vi "WS1050_RFFE_ST Scope Ver1.3.vi"(0 "RFFE PIC":refnum<visa-resource-name>="COM7", 1 "A3643A GPIB":refnum<visa-resource-name>="GPIB1::6::INSTR", 3 "LOT#":string="16VNB", 4 "WAFER#":string="11", 5 "DUT SN":string="SN001R5", 7 "error in (no error)":errorcluster, 8 "Scope USB":refnum<visa-resource-name>="USB0::0x0699::0x0405::C010240::INSTR", 9 "GROUP":string="LEG1-Lord", 12 "path":path=path "C:/Andy/WS1050/ST Test/SN01", 13 "RFT Path":path=path "C:/Andy/WS1050/ST Test", 14 "Start":bool=TRUE, 15 "Stop Loop":bool, 16 "Initilize RFFE ?":bool, 17 "stop":bool=TRUE, 20 "Scope\nSet Up":bool, 22 "Comment":string) -> (10 "RFFE PIC 2":refnum<visa-resource-name>="COM7", 18 "ST Data Out":string[](array[string])=["824.709800E-9", "99.100000E+36", "14.400000E-3", "99.100000E+36", "687.070300E-9", "14.000000E-3", "991.902900E-9", "99.100000E+36", "30.800000E-3", "99.100000E+36", "729.561600E-9", "28.400000E-3", "794.023400E-9", "99.100000E+36", "66.000000E-3", "99.100000E+36", "698.320300E-9", "64.000000E-3", "677.011700E-9", "99.100000E+36", "172.000000E-3", "99.100000E+36", "781.972700E-9", "168.000000E-3", "1.047500E-6", "99.100000E+36", "252.000000E-3", "99.100000E+36", "806.324900E-9", "248.000000E-3", "1.166000E-6", "99.100000E+36", "384.000000E-3", "99.100000E+36", "800.507800E-9", "372.000000E-3", "3.559500E-6", "99.100000E+36", "536.000000E-3", "99.100000E+36", "804.648400E-9", "512.000000E-3", "2.976000E-6", "99.100000E+36", "664.000000E-3", "99.100000E+36", "794.980500E-9", "640.000000E-3", "1.596500E-6", "99.100000E+36", "792.000000E-3", "99.100000E+36", "835.996100E-9", "768.000000E-3", "3.144000E-6", "99.100000E+36", "912.000000E-3", "99.100000E+36", "849.980500E-9", "880.000000E-3", "1.416700E-6", "99.100000E+36", "1.000000E+0", "99.100000E+36", "864.023400E-9", "960.000000E-3", "1.295500E-6", "99.100000E+36", "1.060000E+0", "99.100000E+36", "858.515600E-9", "1.020000E+0", "1.204000E-6", "99.100000E+36", "1.080000E+0", "99.100000E+36", "934.023400E-9", "1.060000E+0", "1.336000E-6", "99.100000E+36", "1.140000E+0", "99.100000E+36", "1.063300E-6", "1.100000E+0", "1.338000E-6", "99.100000E+36", "1.160000E+0", "99.100000E+36", "1.149500E-6", "1.140000E+0", "1.280000E-6", "99.100000E+36", "1.200000E+0", "99.100000E+36", "1.149300E-6", "1.160000E+0", "1.380000E-6", "99.100000E+36", "1.200000E+0", "99.100000E+36", "1.173000E-6", "1.160000E+0", "1.408000E-6", "99.100000E+36", "1.220000E+0", "99.100000E+36", "1.194000E-6", "1.180000E+0", "1.215000E-6", "99.100000E+36", "70.000000E-3", "99.100000E+36", "1.033300E-6", "68.000000E-3", "2.179200E-6", "99.100000E+36", "170.000000E-3", "99.100000E+36", "1.326500E-6", "158.000000E-3", "1.427300E-6", "99.100000E+36", "316.000000E-3", "99.100000E+36", "1.133000E-6", "308.000000E-3", "1.174000E-6", "99.100000E+36", "680.000000E-3", "99.100000E+36", "915.325500E-9", "620.000000E-3", "1.356000E-6", "99.100000E+36", "920.000000E-3", "99.100000E+36", "1.156000E-6", "880.000000E-3", "1.310000E-6", "99.100000E+36", "960.000000E-3", "99.100000E+36", "1.476500E-6", "980.000000E-3", "1.482000E-6", "99.100000E+36", "1.080000E+0", "99.100000E+36", "1.526000E-6", "1.060000E+0", "1.539500E-6", "99.100000E+36", "1.140000E+0", "99.100000E+36", "1.666000E-6", "1.120000E+0", "1.567000E-6", "99.100000E+36", "1.160000E+0", "99.100000E+36", "1.768000E-6", "1.160000E+0", "1.520000E-6", "99.100000E+36", "1.200000E+0", "99.100000E+36", "1.804000E-6", "1.160000E+0", "1.515000E-6", "99.100000E+36", "1.200000E+0", "99.100000E+36", "1.898000E-6", "1.180000E+0", "1.498000E-6", "99.100000E+36", "1.220000E+0", "99.100000E+36", "1.858000E-6", "1.220000E+0", "1.449000E-6", "99.100000E+36", "1.220000E+0", "99.100000E+36", "1.870000E-6", "1.200000E+0", "1.458500E-6", "99.100000E+36", "1.220000E+0", "99.100000E+36", "1.860000E-6", "1.200000E+0", "1.428500E-6", "99.100000E+36", "1.220000E+0", "99.100000E+36", "1.870000E-6", "1.200000E+0", "1.350000E-6", "99.100000E+36", "1.200000E+0", "99.100000E+36", "1.918500E-6", "1.220000E+0", "1.468500E-6", "99.100000E+36", "1.220000E+0", "99.100000E+36", "1.938700E-6", "1.220000E+0", "1.390000E-6", "99.100000E+36", "1.200000E+0", "99.100000E+36", "1.917500E-6", "1.200000E+0", "634.023400E-9", "99.100000E+36", "46.000000E-3", "99.100000E+36", "1.470000E-6", "40.000000E-3", "1.126000E-6", "99.100000E+36", "84.000000E-3", "99.100000E+36", "1.137000E-6", "84.000000E-3", "1.103700E-6", "99.100000E+36", "238.000000E-3", "99.100000E+36", "1.126200E-6", "226.000000E-3", "1.091000E-6", "99.100000E+36", "512.000000E-3", "99.100000E+36", "1.010000E-6", "480.000000E-3", "3.414000E-6", "99.100000E+36", "760.000000E-3", "99.100000E+36", "949.980500E-9", "700.000000E-3", "1.376000E-6", "99.100000E+36", "940.000000E-3", "99.100000E+36", "1.268000E-6", "920.000000E-3", "1.268000E-6", "99.100000E+36", "1.020000E+0", "99.100000E+36", "1.278000E-6", "980.000000E-3", "1.294000E-6", "99.100000E+36", "1.060000E+0", "99.100000E+36", "1.334000E-6", "1.060000E+0", "1.488000E-6", "99.100000E+36", "1.160000E+0", "99.100000E+36", "1.448000E-6", "1.120000E+0", "1.515000E-6", "99.100000E+36", "1.200000E+0", "99.100000E+36", "1.534000E-6", "1.160000E+0", "1.516000E-6", "99.100000E+36", "1.240000E+0", "99.100000E+36", "1.628000E-6", "1.220000E+0", "1.602000E-6", "99.100000E+36", "1.280000E+0", "99.100000E+36", "1.557000E-6", "1.240000E+0", "1.610000E-6", "99.100000E+36", "1.300000E+0", "99.100000E+36", "1.637500E-6", "1.260000E+0", "1.580000E-6", "99.100000E+36", "1.300000E+0", "99.100000E+36", "1.724000E-6", "1.280000E+0", "1.611000E-6", "99.100000E+36", "1.320000E+0", "99.100000E+36", "1.722000E-6", "1.280000E+0", "1.611000E-6", "99.100000E+36", "1.320000E+0", "99.100000E+36", "1.770000E-6", "1.300000E+0", "1.608000E-6", "99.100000E+36", "1.320000E+0", "99.100000E+36", "1.780000E-6", "1.300000E+0", "1.601000E-6", "99.100000E+36", "1.320000E+0", "99.100000E+36", "1.795000E-6", "1.300000E+0"], 19 "ST Header Out":string[](array[string]), 21 "Status":string="Idle....", 24 "Scope USB out":refnum<visa-resource-name>="USB0::0x0699::0x0405::C010240::INSTR", 25 "A3643A Out":refnum<visa-resource-name>="GPIB1::6::INSTR", 27 "error out":errorcluster)   [LabVIEW 2012]
uses:
  <instrlib>/Tektronix DPO MSO 2000 4000 Series/Tektronix DPO MSO 2000 4000 Series.lvlib
panel:
  in  "Save ST Data":bool
  in  "WS1050 C3L Cmd":string[](array[string])=["074301", "074300", "074302", "074300", "074304", "074300", "074308", "074300", "07430C", "074300", "074310", "074300", "074314", "074300", "074318", "074300", "07431C", "074300", "074320", "074300", "074324", "074300", "074328", "074300", "07432C", "074300", "074330", "074300", "074334", "074300", "074338", "074300", "074339", "074300", "07433B", "074300"]
  in  "C3L":string[](array[string])=["C3_S0F1_ON", "C3_S0F1_OFF", "C3_S0F2_ON", "C3_S0F2_OFF", "C3_S1_ON", "C3_S1_OFF", "C3_S2_ON", "C3_S2_OFF", "C3_S3_ON", "C3_S3_OFF", "C3_S4_ON", "C3_S4_OFF", "C3_S5_ON", "C3_S5_OFF", "C3_S6_ON", "C3_S6_OFF", "C3_S7_ON", "C3_S7_OFF", "C3_S8_ON", "C3_S8_OFF", "C3_S9_ON", "C3_S9_OFF", "C3_S10_ON", "C3_S10_OFF", "C3_S11_ON", "C3_S11_OFF", "C3_S12_ON", "C3_S12_OFF", "C3_S13_ON", "C3_S13_OFF", "C3_S14_ON", "C3_S14_OFF", "C3_S14F1_ON", "C3_S14F1_OFF", "C3_S14F12_ON", "C3_S14F12_OFF"]
  in  "C2L":string[](array[string])=["C2_S0F1_ON", "C2_S0F1_OFF", "C2_S0F2_ON", "C2_S0F2_OFF", "C2_S1_ON", "C2_S1_OFF", "C2_S2_ON", "C2_S2_OFF", "C2_S3_ON", "C2_S3_OFF", "C2_S4_ON", "C2_S4_OFF", "C2_S5_ON", "C2_S5_OFF", "C2_S6_ON", "C2_S6_OFF", "C2_S7_ON", "C2_S7_OFF", "C2_S8_ON", "C2_S8_OFF", "C2_S9_ON", "C2_S9_OFF", "C2_S10_ON", "C2_S10_OFF", "C2_S11_ON", "C2_S11_OFF", "C2_S12_ON", "C2_S12_OFF", "C2_S13_ON", "C2_S13_OFF", "C2_S14_ON", "C2_S14_OFF", "C2_S14F1_ON", "C2_S14F1_OFF", "C2_S14F12_ON", "C2_S14F12_OFF"]
  in  "WS1050 C2L Cmd":string[](array[string])=["074201", "074200", "074202", "074200", "074204", "074200", "074208", "074200", "07420C", "074200", "074210", "074200", "074214", "074200", "074218", "074200", "07421C", "074200", "074220", "074200", "074224", "074200", "074228", "074200", "07422C", "074200", "074230", "074200", "074234", "074200", "074238", "074200", "074239", "074200", "07423B", "074200"]
  in  "WS1050 Cmd":string[](array[string])=["074101", "074100", "074102", "074100", "074104", "074108", "07410C", "074110", "074114", "074118", "07411C", "074120", "074124", "074128", "07412C", "074130", "074134", "074138", "074139", "07413B", "074139", "074138", "074134", "074130", "07412C", "074128", "074124", "074120", "07411C", "074118", "074114", "074110", "07410C", "074108", "074104", "074100", "074201", "074200", "074202", "074200", "074204", "074208", "07420C", "074210", "074214", "074218", "07421C", "074220", "074224", "074228", "07422C", "074230", "074234", "074238", "074239", "07423B", "074239", "074238", "074234", "074230", "07422C", "074228", "074224", "074220", "07421C", "074218", "074214", "074210", "07420C", "074208", "074204", "074200", "074301", "074300", "074302", "074300", "074304", "074308", "07430C", "074310", "074314", "074318", "07431C", "074320", "074324", "074328", "07432C", "074330", "074334", "074338", "074339", "07433B", "074339", "074338", "074334", "074330", "07432C", "074328", "074324", "074320", "07431C", "074318", "074314", "074310", "07430C", "074308", "074304", "074300"]
  in  "WS1050 Name":string[](array[string])=["C1L_S0F1_ON", "C1L_S0F1_OFF", "C1L_S0F2_ON", "C1L_S0F2_OFF", "C1L_S1_UP", "C1L_S2_UP", "C1L_S3_UP", "C1L_S4_UP", "C1L_S5_UP", "C1L_S6_UP", "C1L_S7_UP", "C1L_S8_UP", "C1L_S9_UP", "C1L_S10_UP", "C1L_S11_UP", "C1L_S12_UP", "C1L_S13_UP", "C1L_S14_UP", "C1L_S14F1_UP", "C1L_S14F12_UP", "C1L_S14F1_DN", "C1L_S14_DN", "C1L_S13_DN", "C1L_S12_DN", "C1L_S11_DN", "C1L_S10_DN", "C1L_S9_DN", "C1L_S8_DN", "C1L_S7_DN", "C1L_S6_DN", "C1L_S5_DN", "C1L_S4_DN", "C1L_S3_DN", "C1L_S2_DN", "C1L_S1_DN", "C1L_ALL_OFF", "C2L_S0F1_ON", "C2L_S0F1_OFF", "C2L_S0F2_ON", "C2L_S0F2_OFF", "C2L_S1_UP", "C2L_S2_UP", "C2L_S3_UP", "C2L_S4_UP", "C2L_S5_UP", "C2L_S6_UP", "C2L_S7_UP", "C2L_S8_UP", "C2L_S9_UP", "C2L_S10_UP", "C2L_S11_UP", "C2L_S12_UP", "C2L_S13_UP", "C2L_S14_UP", "C2L_S14F1_UP", "C2L_S14F12_UP", "C2L_S14F1_DN", "C2L_S14_DN", "C2L_S13_DN", "C2L_S12_DN", "C2L_S11_DN", "C2L_S10_DN", "C2L_S9_DN", "C2L_S8_DN", "C2L_S7_DN", "C2L_S6_DN", "C2L_S5_DN", "C2L_S4_DN", "C2L_S3_DN", "C2L_S2_DN", "C2L_S1_DN", "C2L_ALL_OFF", "C3L_S0F1_ON", "C3L_S0F1_OFF", "C3L_S0F2_ON", "C3L_S0F2_OFF", "C3L_S1_UP", "C3L_S2_UP", "C3L_S3_UP", "C3L_S4_UP", "C3L_S5_UP", "C3L_S6_UP", "C3L_S7_UP", "C3L_S8_UP", "C3L_S9_UP", "C3L_S10_UP", "C3L_S11_UP", "C3L_S12_UP", "C3L_S13_UP", "C3L_S14_UP", "C3L_S14F1_UP", "C3L_S14F12_UP", "C3L_S14F1_DN", "C3L_S14_DN", "C3L_S13_DN", "C3L_S12_DN", "C3L_S11_DN", "C3L_S10_DN", "C3L_S9_DN", "C3L_S8_DN", "C3L_S7_DN", "C3L_S6_DN", "C3L_S5_DN", "C3L_S4_DN", "C3L_S3_DN", "C3L_S2_DN", "C3L_S1_DN", "C3L_ALL_OFF"]
  in  "WS1050 C1L Cmd":string[](array[string])=["074101", "074100", "074102", "074100", "074104", "074100", "074108", "074100", "07410C", "074100", "074110", "074100", "074114", "074100", "074118", "074100", "07411C", "074100", "074120", "074100", "074124", "074100", "074128", "074100", "07412C", "074100", "074130", "074100", "074134", "074100", "074138", "074100", "074139", "074100", "07413B", "074100"]
  in  "C1L":string[](array[string])=["C1_S0F1_ON", "C1_S0F1_OFF", "C1_S0F2_ON", "C1_S0F2_OFF", "C1_S1_ON", "C1_S1_OFF", "C1_S2_ON", "C1_S2_OFF", "C1_S3_ON", "C1_S3_OFF", "C1_S4_ON", "C1_S4_OFF", "C1_S5_ON", "C1_S5_OFF", "C1_S6_ON", "C1_S6_OFF", "C1_S7_ON", "C1_S7_OFF", "C1_S8_ON", "C1_S8_OFF", "C1_S9_ON", "C1_S9_OFF", "C1_S10_ON", "C1_S10_OFF", "C1_S11_ON", "C1_S11_OFF", "C1_S12_ON", "C1_S12_OFF", "C1_S13_ON", "C1_S13_OFF", "C1_S14_ON", "C1_S14_OFF", "C1_S14F1_ON", "C1_S14F1_OFF", "C1_S14F12_ON", "C1_S14F12_OFF"]
  in  "milliseconds to wait":u32=100
  in  "Bandwidth (0: FULL)":u16(ring)=3 items=["FULL", "250 MHz", "150 MHz", "20 MHz"]
  out "Test Program Name":string=" WS1040 ST Test Program SubVI Ver1.3"
  out "dt":dbl=1e-08
  in  "Timebase":dbl=0.0001
  in  "RFFE Action":i32(ring)=2 items=["-", "Charge Pump Off", "Charge Pump On", "-", "Charge Pump to 40V", "Charge Pump to 35V", "Trim Code 26", "Trim Code 30", "Trim Code 32", "Trim Code 33", "Trim Code 42", "Trim Code 44", "Trim Code 46", "Trim Code 48", "Trim Code 49", "Trim Code 50", "All Drivers Off", "All Drivers On", "Reg1 On", "Reg2 On", "Reg3 On", "Reg4 On"]
  in  "RFFE Action":bool
  in  "Closing Cheetah function calls":i32(listbox)
  # "***Please do not remove***\nCompany:  WiSpry Inc\nCreated by:  Andy V Tran\nDate:  07/25/2013"
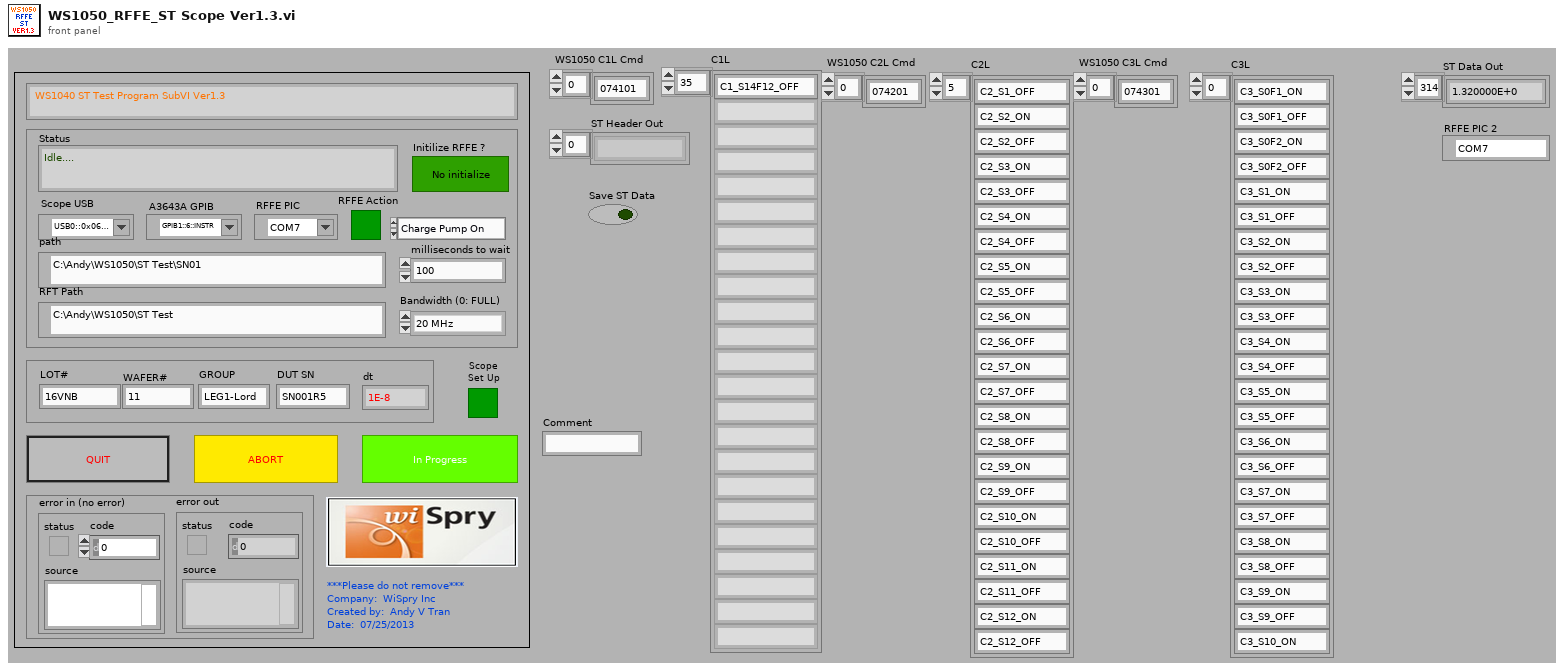
[diagram p1: front panel]
types:
  T1 = enum16{"open", "replace", "create", "open or create", "replace or create", "replace or create with confirmation"}
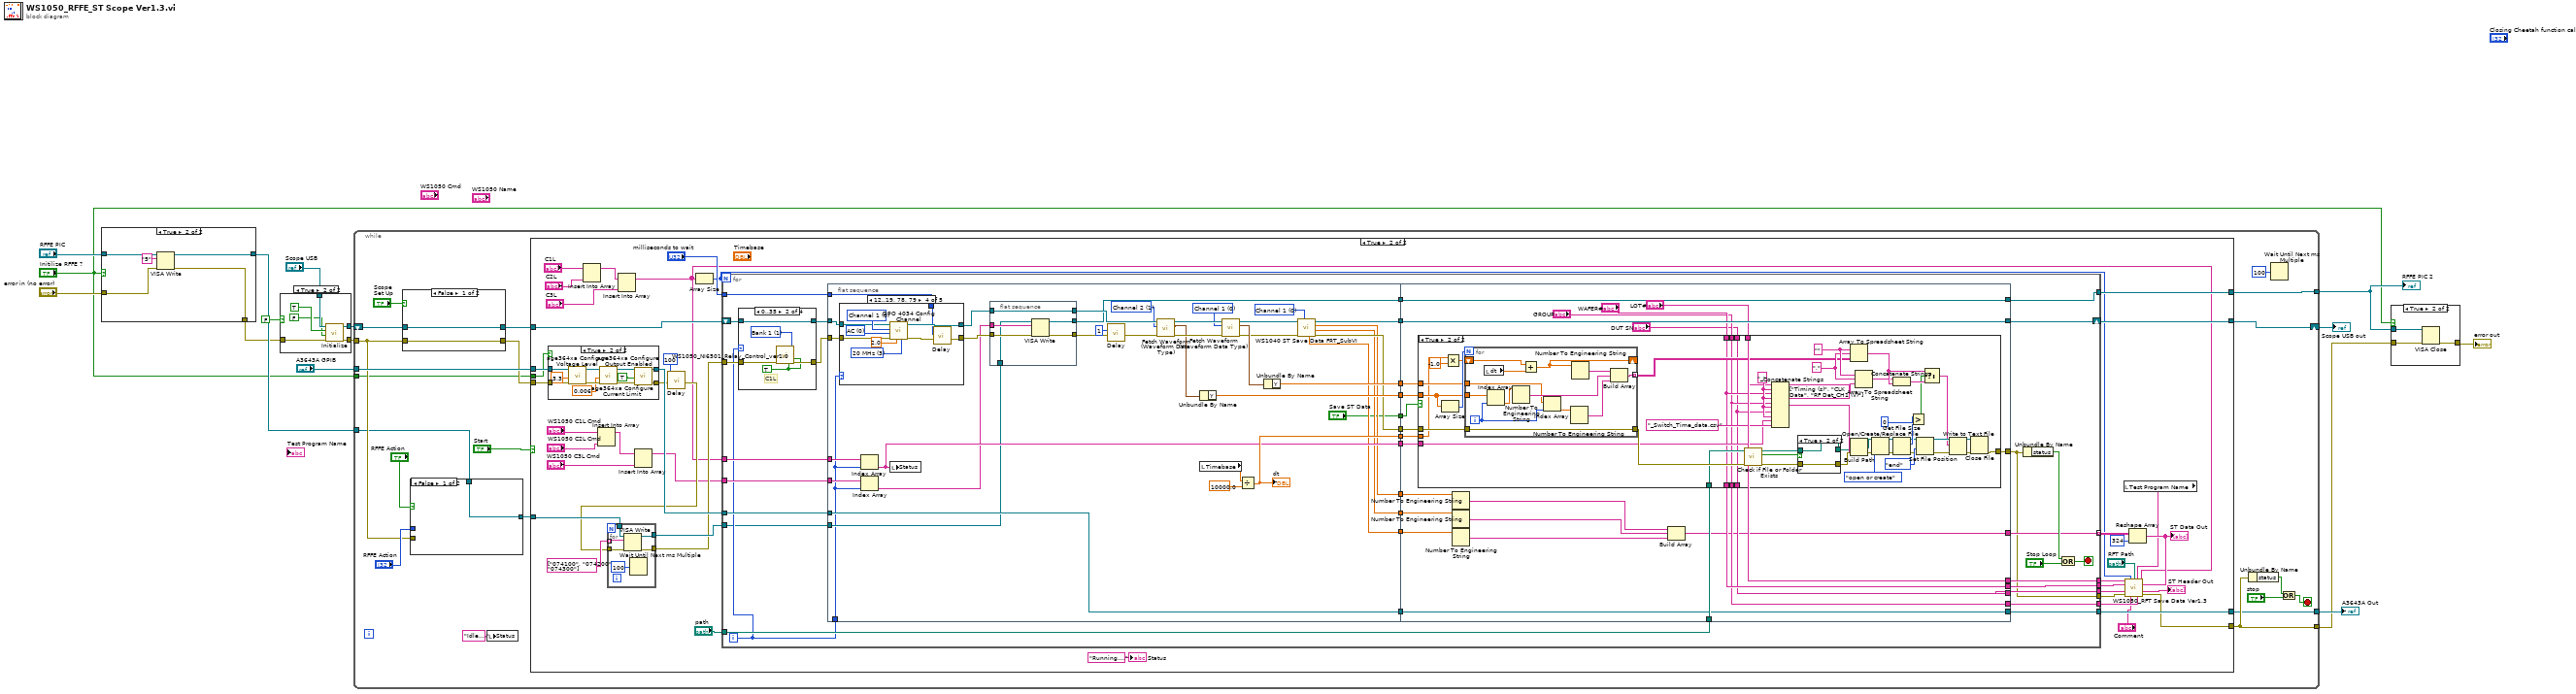
[diagram p0: block diagram]
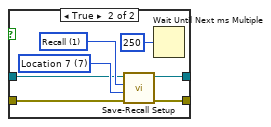
[diagram p3: hidden frame]
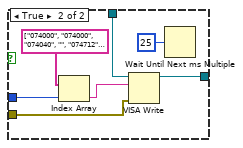
[diagram p4: hidden frame]
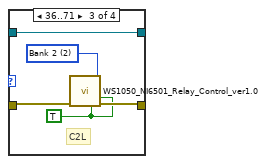
[diagram p8: hidden frame]
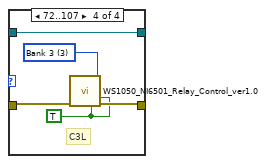
[diagram p9: hidden frame]
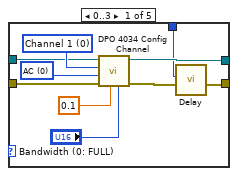
[diagram p10: hidden frame]
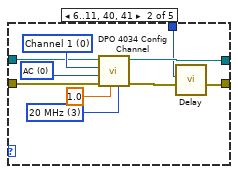
[diagram p11: hidden frame]
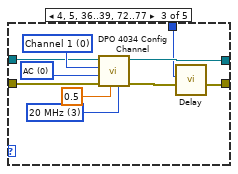
[diagram p12: hidden frame]
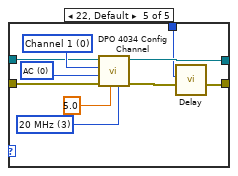
[diagram p13: hidden frame]
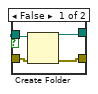
[diagram p15: hidden frame]
diagram:
  n1 = case shown="True" "Initilize RFFE ?" {
    tunnel: [w17 w19] -> w3
    tunnel: "error in (no error)" -> [w17 w20]
    tunnel: "RFFE PIC" -> [w16 w22]
    tunnel: [w16 w18] -> w5
    frame False {
    }
    frame True {
      n2 = VISA Write(VISA resource name=w22, write buffer="5", error in (no error)=w20) -> (VISA resource name out=w18:refnum<visa-resource-name>, error out=w19:errorcluster)  [unwired: 1 out]
    }
  }
  n3 = case shown="True" FALSE {
    tunnel: [w24 w30] -> w9
    tunnel: [w23 w29] -> w8
    tunnel: "Scope USB" -> [w23 w28]
    tunnel: w3 -> [w24 w25]
    frame False {
    }
    frame True {
      n4 = call <instrlib>:"Initialize.vi"("error in (no error)"=w25, "Reset (True)"=FALSE, "ID Query (True)"=TRUE, "VISA resource name"=w28) -> ("error out"=w30:errorcluster, "VISA resource name out"=w29:refnum<visa-resource-name>)  [unwired: 6 in]
    }
  }
  n5 = while {
    tunnel: [w43] -> w10
    tunnel: w9 -> [w34]
    tunnel: "A3643A GPIB" -> [w44]
    tunnel: [w42] -> w14
    shift-right: [w37] -> w11
    shift-left: w8 -> [w40]
    tunnel: w5 -> [w33]
    tunnel: [w35] -> w4
    tunnel: "Initilize RFFE ?" -> [w31]
    stop <- w51 stop-if-true
    n6 = case shown="False" "Scope\nSet Up" {
      tunnel: w34 -> [w53 w57]
      tunnel: [w53 w56] -> w38
      tunnel: w40 -> [w52 w55]
      tunnel: [w52 w54] -> w39
      frame False {
      }
      frame True {
        w58 = u16 7 items=["Location 1"=1, "Location 2"=2, "Location 3"=3, "Location 4"=4, "Location 5"=5, "Location 6"=6, "Location 7"=7, "Location 8"=8, "Location 9"=9, "Location 10"=10] ("Memory Location (1: Location 1)")
        w59 = u16 1 items=["Save", "Recall"] ("Operation (0: Save)")
        n7 = call <instrlib>:"Save-Recall Setup.vi"("error in (no error)"=w57, "Memory Location (1: Location 1)"=w58, "Operation (0: Save)"=w59, "VISA resource name"=w55) -> ("error out"=w56:errorcluster, "VISA resource name out"=w54:refnum<visa-resource-name>)  [unwired: 6 in]
        n8 = Wait Until Next ms Multiple(millisecond multiple=u32 250) -> ()  [unwired: 1 out]
      }
    }
    n9 = case shown="False" "RFFE Action" {
      tunnel: "RFFE Action" -> [_ w67]
      tunnel: w34 -> [_ w65]
      tunnel: w33 -> [w61 w64]
      tunnel: [w61 w63] -> w32
      frame False {
      }
      frame True {
        n10 = Index Array(array=string[] ["074000", "074000", "074040", "", "074712", "07470B"], index=w67) -> (element=w62:string)
        n11 = VISA Write(VISA resource name=w64, write buffer=w62, error in (no error)=w65) -> (VISA resource name out=w63:refnum<visa-resource-name>)  [unwired: 2 out]
        n12 = Wait Until Next ms Multiple(millisecond multiple=u32 25) -> ()  [unwired: 1 out]
      }
    }
    n13 = local write "Status"("Idle...." ("Status")) -> ()
    n14 = case shown="True" "Start" {
      tunnel: [w72 w109] -> w37
      tunnel: w39 -> [w72 w108]
      tunnel: w38 -> [w71 w113]
      tunnel: w44 -> [w70 w112]
      tunnel: [w70 w103] -> w42
      tunnel: [w71 w101] -> w43
      tunnel: [w69 w91] -> w35
      tunnel: w32 -> [w69 w87]
      tunnel: w31 -> [_ w85]
      frame False {
      }
      frame True {
        n15 = case shown="True" w85 {
          tunnel: w113 -> [w115 w127]
          tunnel: w112 -> [w116 w126]
          tunnel: [w116 w118] -> w111
          tunnel: [w115 w117] -> w107
          frame False {
          }
          frame True {
            n16 = call "age364xa Configure Voltage Level.vi"("error in (no error)"=w127, "Level (0.0 Volts)"=3.3, "VISA session"=w126) -> ("error out"=w124:errorcluster, "dup VISA session"=w122:refnum<visa-resource-name>)  [unwired: 7 in]
            n17 = call "age364xa Configure Current Limit.vi"("error in (no error)"=w124, "Current Limit (0.0 Amps)"=0.006, "VISA session"=w122) -> ("error out"=w123:errorcluster, "dup VISA session"=w121:refnum<visa-resource-name>)  [unwired: 7 in]
            n18 = call "age364xa Configure Output Enabled.vi"("error in (no error)"=w123, "Output Enabled (F: Off)"=TRUE, "VISA session"=w121) -> ("error out"=w117:errorcluster, "dup VISA session"=w118:refnum<visa-resource-name>)  [unwired: 7 in]
          }
        }
        n19 = Insert Into Array(array="C1L", new element="C2L") -> (w77:string[])  [unwired: 1 in]
        n20 = Insert Into Array(array="WS1050 C1L Cmd", new element="WS1050 C2L Cmd") -> (w82:string[])  [unwired: 1 in]
        n21 = Insert Into Array(array=w77, new element="C3L") -> (w75:string[])  [unwired: 1 in]
        n22 = Insert Into Array(array=w82, new element="WS1050 C3L Cmd") -> (w80:string[])  [unwired: 1 in]
        n23 = call "Delay.vi"("error in (no error)"=w107, "milliseconds to wait"=u32 100) -> ("error out"=w86:errorcluster)  [unwired: 9 in]
        n24 = for {
          tunnel: w86 -> [w133]
          tunnel: w87 -> [w132]
          tunnel: [w131] -> w90
          tunnel: [w130] -> w89
          tunnel: string[] ["074100", "074200", "074300"] -> [w128] mode=indexing
          n25 = VISA Write(VISA resource name=w132, write buffer=w128, error in (no error)=w133) -> (VISA resource name out=w131:refnum<visa-resource-name>, error out=w130:errorcluster)  [unwired: 1 out]
          n26 = Wait Until Next ms Multiple(millisecond multiple=u32 100) -> ()  [unwired: 1 out]
        }
        n27 = Array Size(array=w75) -> (size(s)=w73:i32)
        n28 = for {
          N: w73 -> [_]
          tunnel: [w136] -> w102
          tunnel: "path" -> [w164]
          tunnel: w111 -> [w156]
          tunnel: [w154] -> w103
          tunnel: w89 -> [w148]
          tunnel: w75 -> [w153]
          tunnel: w80 -> [w151]
          tunnel: "milliseconds to wait" -> [w150]
          shift-right: [w149] -> w109
          shift-left: w108 -> [w146]
          tunnel: [w143] -> w100
          tunnel: [w142] -> w99
          tunnel: [w141] -> w98
          tunnel: [w140] -> w96
          tunnel: [w139] -> w95 mode=indexing
          tunnel: w90 -> [w138]
          tunnel: [w135] -> w91
          i -> [w144]
          stop <- w166 stop-if-true
          n29 = case shown="0..35" w144 {
            tunnel: w148 -> [w169 w175 w179 w184]
            tunnel: [w169 w174 w180 w185] -> w147
            tunnel: w146 -> [w170 w173 w178 w183]
            tunnel: [w170 w173 w178 w183] -> w145
            frame 108, Default {
            }
            frame 0..35 {
              w171 = TRUE ("Relay_ 10")
              w172 = u16 1 items=["All Off", "Bank 1", "Bank 2", "Bank 3"] ("Ring")
              # "C1L"
              n30 = call "WS1050_NI6501_Relay_Control_ver1.0.vi"("Ring"=w172, "Relay_ 11"=w171, "error in (no error)"=w175, "Relay_ 10"=w171) -> ("error out"=w174:errorcluster)  [unwired: 2 in, 9 out]
            }
            frame 36..71 {
              w176 = TRUE ("Relay_ 10")
              w177 = u16 2 items=["All Off", "Bank 1", "Bank 2", "Bank 3"] ("Ring")
              # "C2L"
              n31 = call "WS1050_NI6501_Relay_Control_ver1.0.vi"("Ring"=w177, "Relay_ 11"=w176, "error in (no error)"=w179, "Relay_ 10"=w176) -> ("error out"=w180:errorcluster)  [unwired: 2 in, 9 out]
            }
            frame 72..107 {
              w181 = TRUE ("Relay_ 10")
              w182 = u16 3 items=["All Off", "Bank 1", "Bank 2", "Bank 3"] ("Ring")
              # "C3L"
              n32 = call "WS1050_NI6501_Relay_Control_ver1.0.vi"("Ring"=w182, "Relay_ 11"=w181, "error in (no error)"=w184, "Relay_ 10"=w181) -> ("error out"=w185:errorcluster)  [unwired: 2 in, 9 out]
            }
          }
          n33 = flat-sequence {
            tunnel: w144 -> [w187]
            tunnel: [w201] -> w165
            tunnel: [w202] -> w163
            tunnel: [w219] -> w162
            tunnel: [w218] -> w161
            tunnel: [w198] -> w160
            tunnel: [w199] -> w159
            tunnel: [w200] -> w158
            tunnel: [w221] -> w157
            tunnel: w156 -> [w220]
            tunnel: [w220] -> w155
            tunnel: w147 -> [w216]
            tunnel: w145 -> [w215]
            tunnel: w153 -> [w213]
            tunnel: [w212] -> w152
            tunnel: w151 -> [w211]
            tunnel: w150 -> [w210]
            tunnel: w138 -> [w197]
            tunnel: [w196] -> w137
            tunnel: ["Save ST Data"] -> w134
            tunnel: [w303] -> w149
            tunnel: w165 -> [w303]
            tunnel: [w302] -> w136
            tunnel: w164 -> [w294]
            tunnel: w163 -> [w301]
            tunnel: w162 -> [w300]
            tunnel: w161 -> [w299]
            tunnel: w160 -> [w295]
            tunnel: w159 -> [w296]
            tunnel: w158 -> [w297]
            tunnel: w157 -> [w298]
            tunnel: w155 -> [w293]
            tunnel: [w293] -> w154
            tunnel: w152 -> [w292]
            tunnel: ["LOT#"] -> w143
            tunnel: [w290] -> w142
            tunnel: [w289] -> w141
            tunnel: [w288] -> w140
            tunnel: [w284] -> w139
            tunnel: w137 -> [w283]
            tunnel: [w283] -> w135
            tunnel: w134 -> [w279]
            frame #0 {
              w191 = u16 0 items=["Channel 1", "Channel 2", "Channel 3", "Channel 4", "Math", "Reference 1", "Reference 2", "Reference 3", "Reference 4"] ("Destination Channel (1: Channel 2)")
              w195 = u16 0 items=["Channel 1", "Channel 2", "Channel 3", "Channel 4", "Math", "Reference 1", "Reference 2", "Reference 3", "Reference 4", "D0", "D1", "D2", "D3", "D4", "D5", "D6", "D7", "D8", "D9", "D10", "D11", "D12", "D13", "D14", "D15", "Amplitude", "Frequency", "Phase", "Normal", "Average", "Maximum Peak Hold", "Minimum Peak Hold"] ("Channel (0: Channel 1)")
              w203 = u16 1 items=["Channel 1", "Channel 2", "Channel 3", "Channel 4", "Math", "Reference 1", "Reference 2", "Reference 3", "Reference 4", "D0", "D1", "D2", "D3", "D4", "D5", "D6", "D7", "D8", "D9", "D10", "D11", "D12", "D13", "D14", "D15", "Amplitude", "Frequency", "Phase", "Normal", "Average", "Maximum Peak Hold", "Minimum Peak Hold"] ("Channel (0: Channel 1)")
              n34 = case shown="12..19, 78, 79" w187 {
                tunnel: w216 -> [w229 w240 w250 w260 w270]
                tunnel: w215 -> [w228 w239 w249 w259 w269]
                tunnel: [w227 w238 w248 w258 w268] -> w214
                tunnel: w210 -> [w224 w235 w245 w255 w265]
                tunnel: [w225 w236 w246 w256 w266] -> w208
                frame 0..3 {
                  w232 = u16 0 items=["Channel 1", "Channel 2", "Channel 3", "Channel 4", "Math", "Reference 1", "Reference 2", "Reference 3", "Reference 4", "Bus 1", "Bus 2"] ("Channel (0: Channel 1)")
                  w231 = u16 0 items=["AC", "DC", "Ground"] ("Vertical Coupling (1: DC)")
                  n35 = call "DPO 4034 Config Channel.vi"("Bandwidth (0: FULL)"="Bandwidth (0: FULL)", "Vertical Range (10.0 V)"=0.1, "error in (no error)"=w229, "Vertical Coupling (1: DC)"=w231, "Channel (0: Channel 1)"=w232, "VISA resource name"=w228) -> ("error out"=w226:errorcluster, "VISA resource name out"=w225:refnum<visa-resource-name>)  [unwired: 4 in]
                  n36 = call "Delay.vi"("error in (no error)"=w226, "milliseconds to wait"=w224) -> ("error out"=w227:errorcluster)  [unwired: 9 in]
                }
                frame 6..11, 40, 41 {
                  w233 = u16 3 items=["FULL", "250 MHz", "150 MHz", "20 MHz"] ("Bandwidth (0: FULL)")
                  w242 = u16 0 items=["Channel 1", "Channel 2", "Channel 3", "Channel 4", "Math", "Reference 1", "Reference 2", "Reference 3", "Reference 4", "Bus 1", "Bus 2"] ("Channel (0: Channel 1)")
                  w241 = u16 0 items=["AC", "DC", "Ground"] ("Vertical Coupling (1: DC)")
                  n37 = call "DPO 4034 Config Channel.vi"("Bandwidth (0: FULL)"=w233, "Vertical Range (10.0 V)"=1.0, "error in (no error)"=w240, "Vertical Coupling (1: DC)"=w241, "Channel (0: Channel 1)"=w242, "VISA resource name"=w239) -> ("error out"=w237:errorcluster, "VISA resource name out"=w236:refnum<visa-resource-name>)  [unwired: 4 in]
                  n38 = call "Delay.vi"("error in (no error)"=w237, "milliseconds to wait"=w235) -> ("error out"=w238:errorcluster)  [unwired: 9 in]
                }
                frame 4, 5, 36..39, 72..77 {
                  w243 = u16 3 items=["FULL", "250 MHz", "150 MHz", "20 MHz"] ("Bandwidth (0: FULL)")
                  w252 = u16 0 items=["Channel 1", "Channel 2", "Channel 3", "Channel 4", "Math", "Reference 1", "Reference 2", "Reference 3", "Reference 4", "Bus 1", "Bus 2"] ("Channel (0: Channel 1)")
                  w251 = u16 0 items=["AC", "DC", "Ground"] ("Vertical Coupling (1: DC)")
                  n39 = call "DPO 4034 Config Channel.vi"("Bandwidth (0: FULL)"=w243, "Vertical Range (10.0 V)"=0.5, "error in (no error)"=w250, "Vertical Coupling (1: DC)"=w251, "Channel (0: Channel 1)"=w252, "VISA resource name"=w249) -> ("error out"=w247:errorcluster, "VISA resource name out"=w246:refnum<visa-resource-name>)  [unwired: 4 in]
                  n40 = call "Delay.vi"("error in (no error)"=w247, "milliseconds to wait"=w245) -> ("error out"=w248:errorcluster)  [unwired: 9 in]
                }
                frame 12..19, 78, 79 {
                  w253 = u16 3 items=["FULL", "250 MHz", "150 MHz", "20 MHz"] ("Bandwidth (0: FULL)")
                  w262 = u16 0 items=["Channel 1", "Channel 2", "Channel 3", "Channel 4", "Math", "Reference 1", "Reference 2", "Reference 3", "Reference 4", "Bus 1", "Bus 2"] ("Channel (0: Channel 1)")
                  w261 = u16 0 items=["AC", "DC", "Ground"] ("Vertical Coupling (1: DC)")
                  n41 = call "DPO 4034 Config Channel.vi"("Bandwidth (0: FULL)"=w253, "Vertical Range (10.0 V)"=2.0, "error in (no error)"=w260, "Vertical Coupling (1: DC)"=w261, "Channel (0: Channel 1)"=w262, "VISA resource name"=w259) -> ("error out"=w257:errorcluster, "VISA resource name out"=w256:refnum<visa-resource-name>)  [unwired: 4 in]
                  n42 = call "Delay.vi"("error in (no error)"=w257, "milliseconds to wait"=w255) -> ("error out"=w258:errorcluster)  [unwired: 9 in]
                }
                frame 22, Default {
                  w263 = u16 3 items=["FULL", "250 MHz", "150 MHz", "20 MHz"] ("Bandwidth (0: FULL)")
                  w272 = u16 0 items=["Channel 1", "Channel 2", "Channel 3", "Channel 4", "Math", "Reference 1", "Reference 2", "Reference 3", "Reference 4", "Bus 1", "Bus 2"] ("Channel (0: Channel 1)")
                  w271 = u16 0 items=["AC", "DC", "Ground"] ("Vertical Coupling (1: DC)")
                  n43 = call "DPO 4034 Config Channel.vi"("Bandwidth (0: FULL)"=w263, "Vertical Range (10.0 V)"=5.0, "error in (no error)"=w270, "Vertical Coupling (1: DC)"=w271, "Channel (0: Channel 1)"=w272, "VISA resource name"=w269) -> ("error out"=w267:errorcluster, "VISA resource name out"=w266:refnum<visa-resource-name>)  [unwired: 4 in]
                  n44 = call "Delay.vi"("error in (no error)"=w267, "milliseconds to wait"=w265) -> ("error out"=w268:errorcluster)  [unwired: 9 in]
                }
              }
              n45 = Index Array(array=w213, index=w187) -> (element=w212:string)
              n46 = Index Array(array=w211, index=w187) -> (element=w209:string)
              n47 = local write "Status"(w212) -> ()
              n48 = flat-sequence {
                tunnel: w214 -> [w276]
                tunnel: [w275] -> w189
                tunnel: w208 -> [w278]
                tunnel: [w278] -> w207
                tunnel: w209 -> [w277]
                tunnel: w197 -> [w274]
                tunnel: [w273] -> w196
                frame #0 {
                  n49 = VISA Write(VISA resource name=w274, write buffer=w277, error in (no error)=w276) -> (VISA resource name out=w273:refnum<visa-resource-name>, error out=w275:errorcluster)  [unwired: 1 out]
                }
              }
              n50 = call "Delay.vi"("error in (no error)"=w189, "milliseconds to wait"=u32 1) -> ("error out"=w190:errorcluster)  [unwired: 9 in]
              n51 = call <instrlib>:"Fetch Waveform (Waveform Data Type).vi"("error in (no error)"=w190, "Channel (0: Channel 1)"=w203, "VISA resource name"=w207) -> ("error out"=w206:errorcluster, "Waveform Data"=w205:waveform(dbl), "VISA resource name out"=w204:refnum<visa-resource-name>)  [unwired: 6 in]
              n52 = Unbundle By Name(w205) -> ("Y"=w219:dbl[])
              n53 = local read "Timebase"() -> (w217:dbl)
              n54 = call <instrlib>:"Fetch Waveform (Waveform Data Type).vi"("error in (no error)"=w206, "Channel (0: Channel 1)"=w195, "VISA resource name"=w204) -> ("error out"=w193:errorcluster, "Waveform Data"=w194:waveform(dbl), "VISA resource name out"=w192:refnum<visa-resource-name>)  [unwired: 6 in]
              n55 = Divide(x=w217, y=10000.0) -> (x/y=w221:dbl)
              "dt" <- w221
              n56 = Unbundle By Name(w194) -> ("Y"=w218:dbl[])
              n57 = call "WS1040 ST Save Data FRT_SubVI.vi"("Destination Channel (1: Channel 2)"=w191, "error in (no error)"=w193, "VISA resource name"=w192) -> ("error out"=w202:errorcluster, "Fall Time Value"=w199:dbl, "Rise Time Value"=w200:dbl, "VISA resource name out"=w201:refnum<visa-resource-name>, "Amp_FT"=w198:dbl)  [unwired: 4 in]
            }
            frame #1 {
              n58 = case shown="True" w279 {
                tunnel: [w304 w325] -> w302
                tunnel: w301 -> [w304 w324]
                tunnel: w300 -> [_ w321]
                tunnel: w299 -> [_ w320]
                tunnel: w298 -> [_ w317]
                tunnel: w294 -> [_ w313]
                tunnel: w292 -> [_ w312]
                tunnel: "LOT#" -> [_ w311]
                tunnel: [w305 w310] -> w290
                tunnel: [w306 w309] -> w289
                tunnel: [w307 w308] -> w288
                tunnel: "WAFER#" -> [w305 w310]
                tunnel: "GROUP" -> [w306 w309]
                tunnel: "DUT SN" -> [w307 w308]
                frame False {
                }
                frame True {
                  w314 = "_" ("string")
                  w349 = ""
                  w348 = ","
                  n59 = Array Size(array=w321) -> (size(s)=w322:i32)
                  n60 = Multiply(x=w317, y=-1.0) -> (x*y=w318:dbl)
                  n61 = for {
                    N: w322 -> [_]
                    tunnel: w321 -> [w360]
                    tunnel: [w362] -> w319 mode=indexing
                    shift-right: [w357] -> _
                    shift-left: w318 -> [w358]
                    tunnel: [w356] -> w323
                    tunnel: w324 -> [w356]
                    tunnel: w320 -> [w355]
                    i -> [w353]
                    n62 = local read "dt"() -> (w354:dbl)
                    n63 = Index Array(array=w360, index=w353) -> (element=w361:dbl)
                    n64 = Number To Engineering String(4:w361) -> (0:w363:string)  [unwired: 3 in]
                    n65 = Add(x=w358, y=w354) -> (x+y=w357:dbl)
                    n66 = Index Array(array=w355, index=w353) -> (element=w365:dbl)
                    n67 = Number To Engineering String(4:w365) -> (0:w364:string)  [unwired: 3 in]
                    n68 = Number To Engineering String(4:w357) -> (0:w359:string)  [unwired: 3 in]
                    n69 = Build Array(w359, w363, w364) -> (w362:string[])
                  }
                  n70 = call <vilib>:"Check if File or Folder Exists.vi"("error in (no error)"=w323, "path"=w313) -> ("error out"=w343:errorcluster, "file or folder exists?"=w347:bool, "dup path"=w342:path)  [unwired: 7 out]
                  n71 = Concatenate Strings(w311, w314, w310, w314, w309, w314, w308, w314, w312, "_Switch_Time_data.csv" ("string")) -> (w345:string)
                  n72 = case shown="True" w347 {
                    tunnel: w343 -> [w366 w371]
                    tunnel: [w368 w371] -> w346
                    tunnel: w342 -> [w369 w370]
                    tunnel: [w367 w370] -> w344
                    frame False {
                      n73 = Create Folder(path (use dialog)=w369, error in=w366) -> (created path=w367:path, error out=w368:errorcluster)  [unwired: 2 out]
                    }
                    frame True {
                    }
                  }
                  n74 = Array To Spreadsheet String(delimiter (Tab)=w348, array=w319, 3:w349) -> (spreadsheet string=w350:string)
                  n75 = Build Path(base path=w344, name or relative path=w345) -> (appended path=w341:path)
                  n76 = Array To Spreadsheet String(delimiter (Tab)=w348, array=string[] ["Timing (s)", "CLK Data", "RF Det_CH1 (V)"] ("Array"), 3:w349) -> (spreadsheet string=w338:string)
                  n77 = Open/Create/Replace File(file path (use dialog)=w341, error in=w346, operation (0:open)=T1."open or create") -> (refnum out=w326:refnum<file>, error out=w330:errorcluster)  [unwired: 4 out]
                  n78 = Concatenate Strings(w338, w350) -> (w339:string)
                  n79 = Get File Size(file=w326, error in=w330) -> (refnum out=w327:refnum<file>, size (in bytes)=w332:i64, 0:w328:errorcluster)
                  n80 = Greater?(x=w332, y=i64 0) -> (0:w334:bool)
                  n81 = Set File Position(refnum=w327, from (0:start)=enum16{"start", "end", "current"}."end", error in=w328) -> (refnum out=w352:refnum<file>, error out=w329:errorcluster)  [unwired: 1 out]
                  n82 = Select(t=w350, s=w334, f=w339) -> (s? t:f=w351:string)
                  n83 = Write to Text File(file (use dialog)=w352, text=w351, error in=w329) -> (refnum out=w336:refnum<file>, error out=w335:errorcluster)  [unwired: 2 out]
                  n84 = Close File(refnum=w336, error in=w335) -> (error out=w325:errorcluster)  [unwired: 1 out]
                }
              }
              n85 = Number To Engineering String(4:w297) -> (0:w287:string)  [unwired: 3 in]
              n86 = Number To Engineering String(4:w296) -> (0:w286:string)  [unwired: 3 in]
              n87 = Number To Engineering String(4:w295) -> (0:w285:string)  [unwired: 3 in]
              n88 = Build Array(w287, w286, w285) -> (w284:string[])
            }
          }
          n89 = Unbundle By Name(w136) -> ("status"=w168:bool)
          n90 = Or(x=w168, y="Stop Loop") -> (x .or. y?=w166:bool)
        }
        n91 = local read "Test Program Name"() -> (w92:string)
        n92 = Reshape Array(w95, 324 ("dimension size")) -> (w93:string[])
        "ST Data Out" <- w93
        n93 = call "WS1050_RFT Save Data Ver1.3.vi"("Lot#"=w100, "Numeric"=w73, "RFT Path"="RFT Path", "Test Program Name"=w92, "output Header"=w75, "Wafer#"=w99, "RFT"=w93, "SN#"=w96, "error in (no error)"=w102, "Comment"="Comment", "Group#"=w98) -> ("ST Header Out"=→"ST Header Out":string[], "error out"=w101:errorcluster)  [unwired: 3 in]
        "Status" <- "Running...." ("Status")
      }
    }
    n94 = Unbundle By Name(w43) -> ("status"=w50:bool)
    n95 = Wait Until Next ms Multiple(millisecond multiple=u32 100) -> ()  [unwired: 1 out]
    n96 = Or(x=w50, y="stop") -> (x .or. y?=w51:bool)
  }
  "Scope USB out" <- w11
  "A3643A Out" <- w14
  "RFFE PIC 2" <- w4
  n97 = case shown="True" "Initilize RFFE ?" {
    tunnel: w10 -> [w372 w375]
    tunnel: [w372 w374] -> w13
    tunnel: w4 -> [_ w373]
    frame False {
    }
    frame True {
      n98 = VISA Close(VISA resource name=w373, error in (no error)=w375) -> (error out=w374:errorcluster)
    }
  }
  "error out" <- w13
